vi "UI.vi"() -> ()   [LabVIEW 2016, in "DR803M4.lvlib"]
uses:
  DR803M4.lvlib
  Global variable/hold variable.vi
  Global variable/input variable.vi
  <vilib>/Utility/config.llb/NI_LVConfig.lvlib
panel:
  out "通讯":bool
  out "单次采样量":u16
  out "版本号":string
  out "留样模式":enum16{"定时留样", "时间等比例", "同步留样", "外控留样", "超标留样"}(ring)
  out "门状态":enum16{"门关", "门开"}(ring)
  out "当前瓶号":u16
  out "采样器状态":enum16{"停止", "运行"}(ring)
  out "采样器进程":i32(listbox)
  out "进程":u16(ring) items=["待机"=1, "采样瓶排空"=2, "采样瓶润洗"=5, "进样"=6, "取样"=8, "取样管排空"=9]
  in  "超标留样浓度设置":bool
  out "error out":errorcluster
  in  "VISA资源名称":refnum<visa-resource-name>
  in  "停止":bool
  in  "启动":bool
  in  "门禁":bool
  in  "远程留样":bool
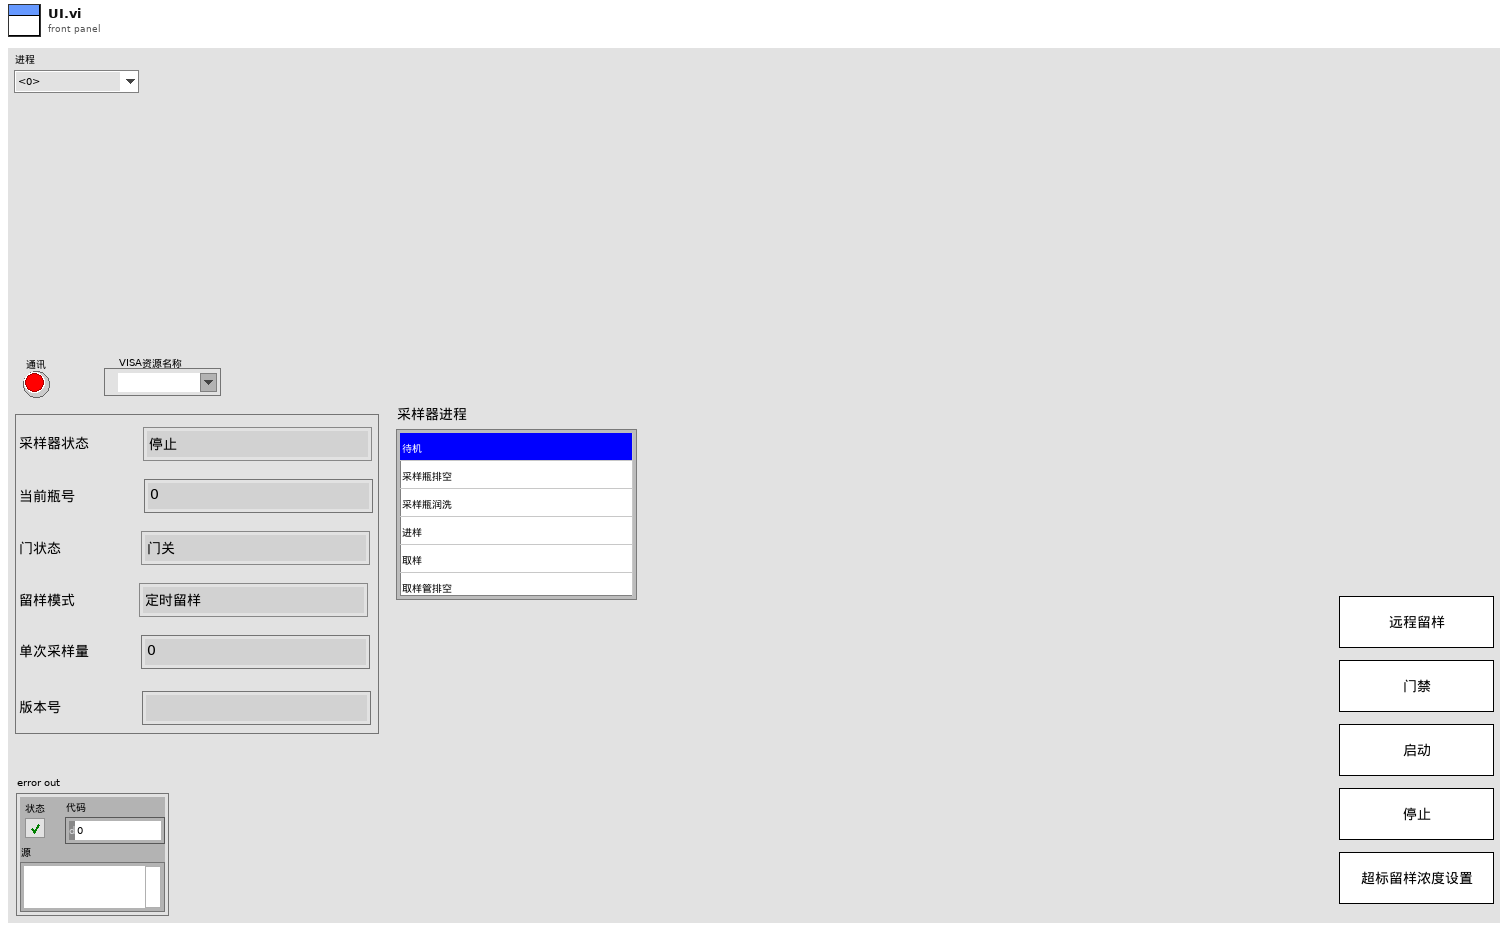
[diagram p1: front panel]
types:
  T1 = cluster{"氨氮超标浓度":dbl, "总磷超标浓度":dbl, "总氮超标浓度":dbl, "CODMn超标浓度":dbl, "CODCr超标浓度":dbl, "PH超标浓度":dbl, "DO超标浓度":dbl, "SPCOND超标浓度":dbl, "浊度超标浓度":dbl, "叶绿素a超标浓度":dbl, "蓝绿藻超标浓度":dbl, "藻密度超标浓度":dbl, "ORP超标浓度":dbl, "COD超标浓度":dbl, "铅超标浓度":dbl, "镉超标浓度":dbl, "铜超标浓度":dbl, "锌超标浓度":dbl, "镍超标浓度":dbl, "锰超标浓度":dbl, "汞超标浓度":dbl}
  T2 = cluster{"确定":bool, "氨氮超标浓度":dbl, "总磷超标浓度":dbl, "总氮超标浓度":dbl, "CODMn超标浓度":dbl, "CODCr超标浓度":dbl, "PH超标浓度":dbl, "DO超标浓度":dbl, "SPCOND超标浓度":dbl, "浊度超标浓度":dbl, "叶绿素a超标浓度":dbl, "蓝绿藻超标浓度":dbl, "藻密度超标浓度":dbl, "ORP超标浓度":dbl, "COD超标浓度":dbl, "铅超标浓度":dbl, "镉超标浓度":dbl, "铜超标浓度":dbl, "锌超标浓度":dbl, "镍超标浓度":dbl, "锰超标浓度":dbl, "汞超标浓度":dbl}
  T3 = typedef "NI_LVConfig.lvlib/Config Data RefNum.ctl" = refnum<k1>
  T4 = cluster{"远程留样":u16, "门禁标志":u16, "门禁密码":u32, "采样器进程":u16, "版本号":string, "启停":u16, "当前瓶号":u16, "采样模式选择":u16, "单次采样量":u16, "时间间隔":u16}
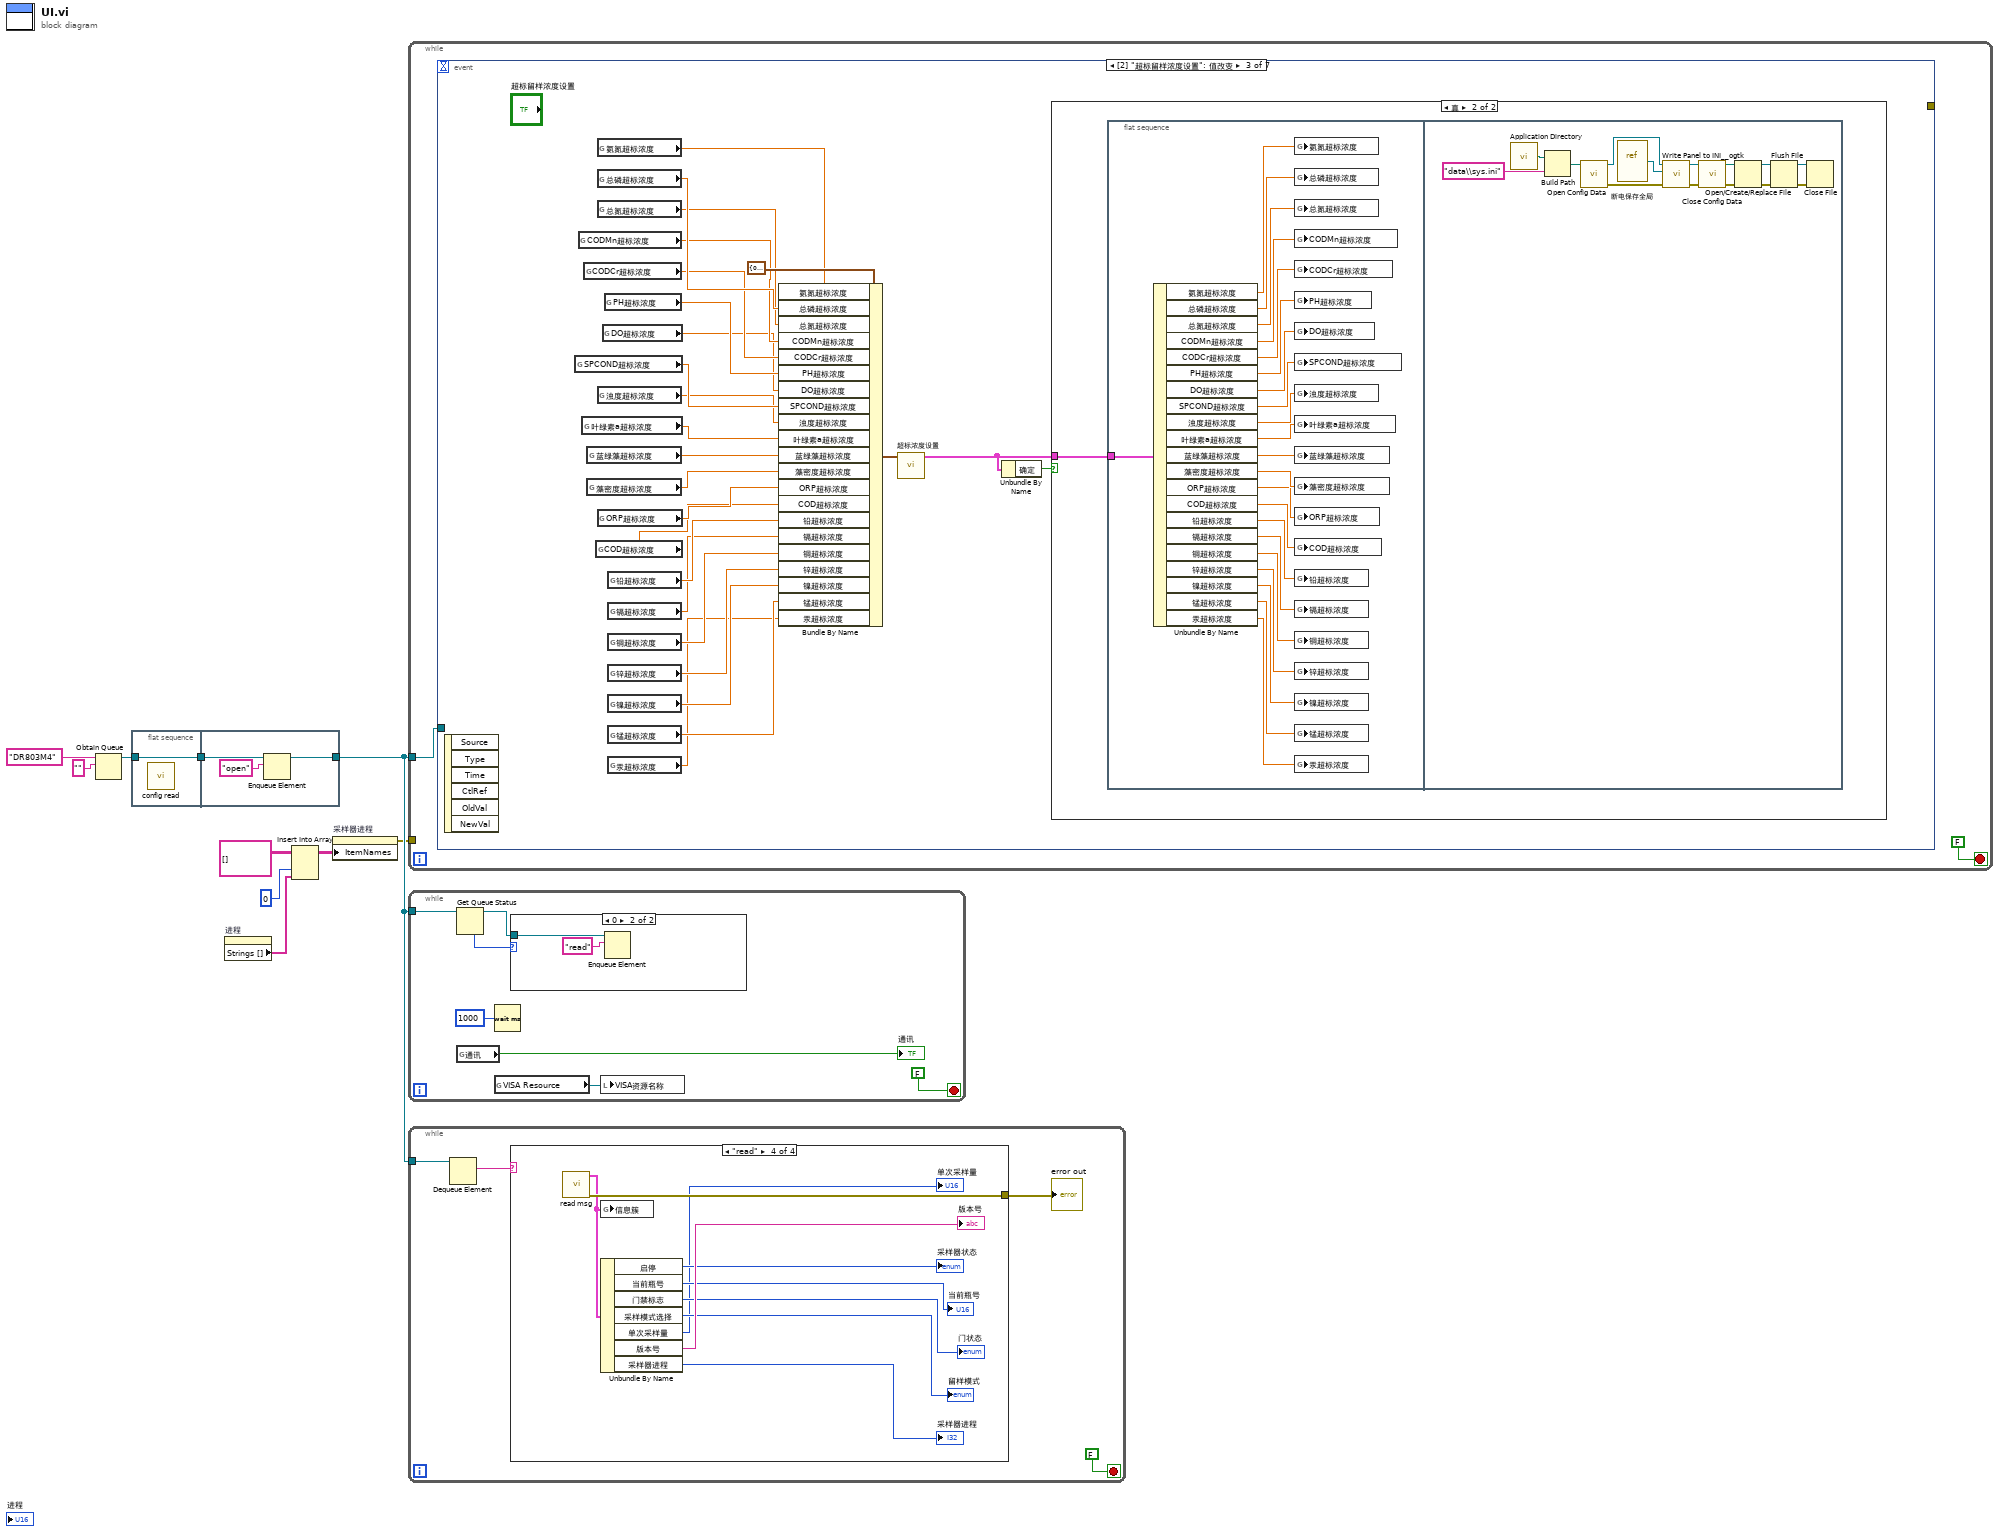
[diagram p0: block diagram]
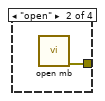
[diagram p4: hidden frame]
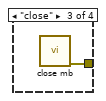
[diagram p5: hidden frame]
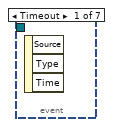
[diagram p6: hidden frame]
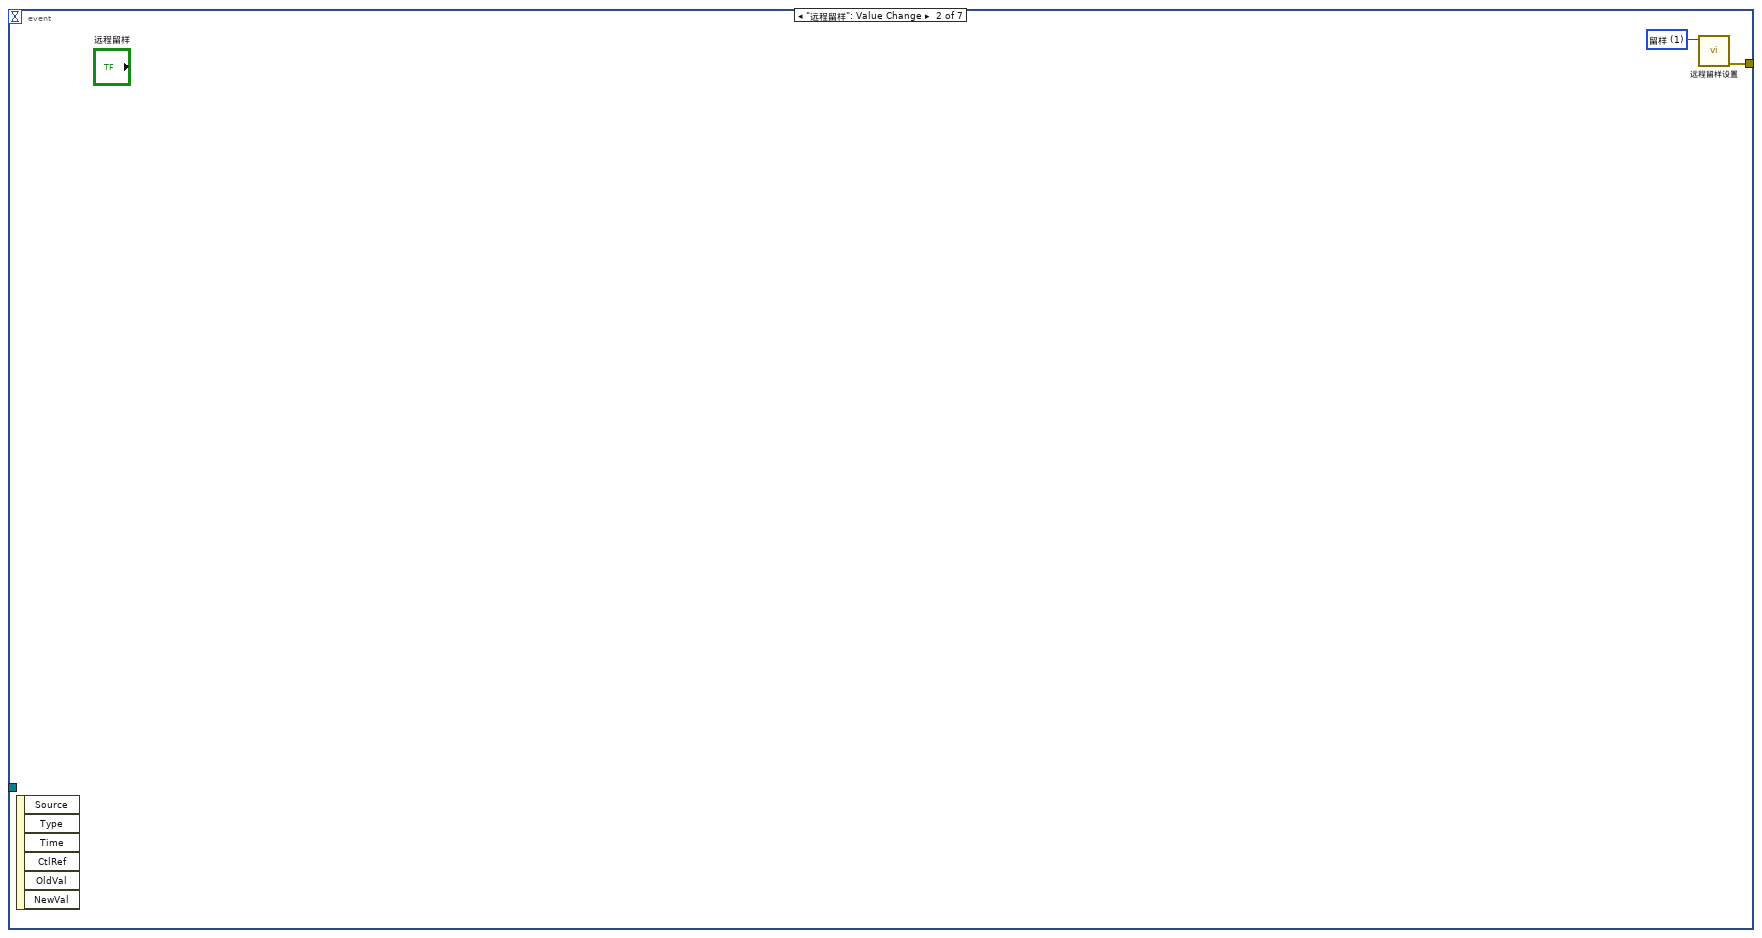
[diagram p7: hidden frame]
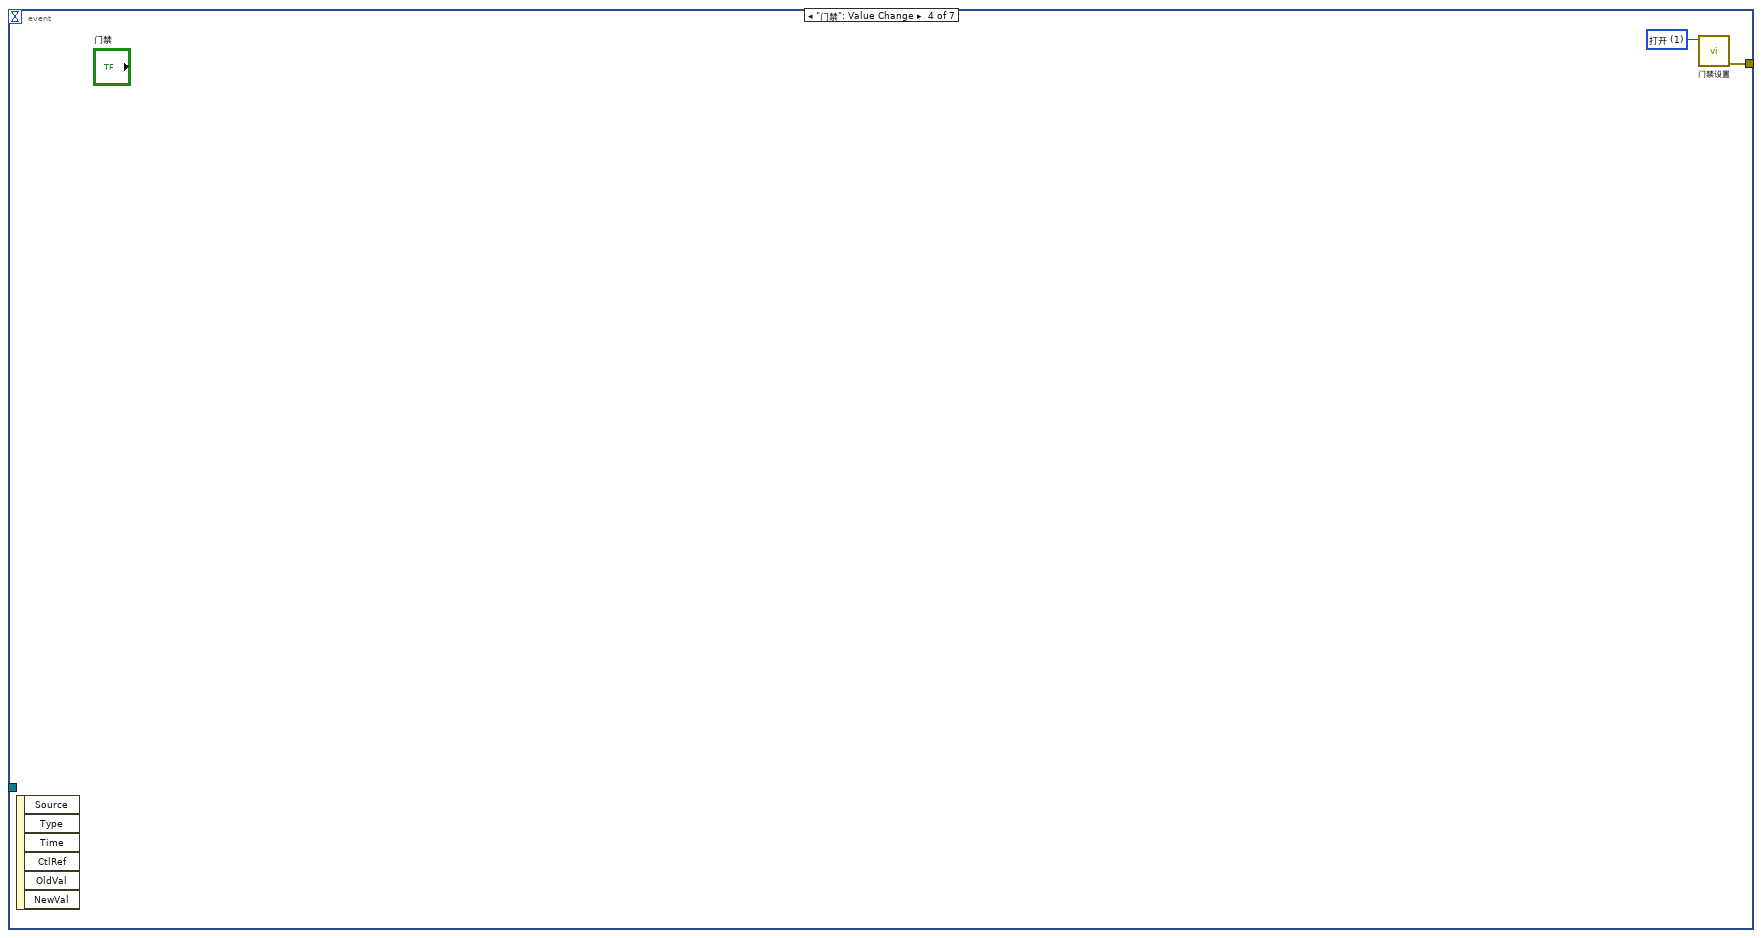
[diagram p9: hidden frame]
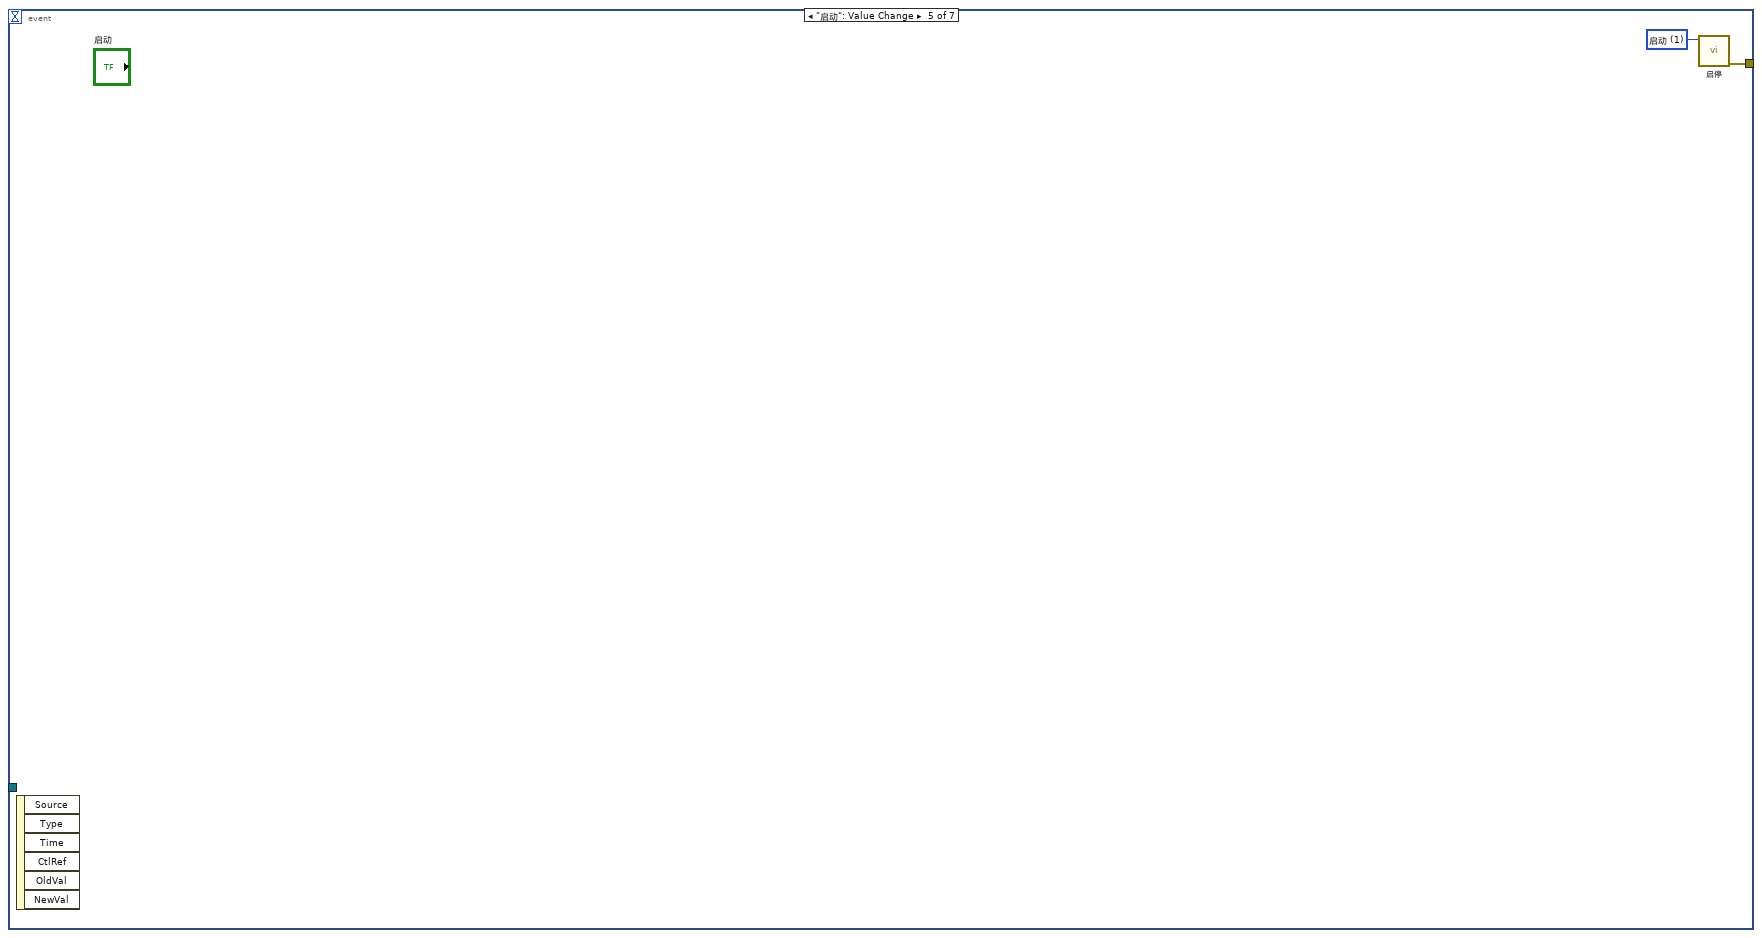
[diagram p10: hidden frame]
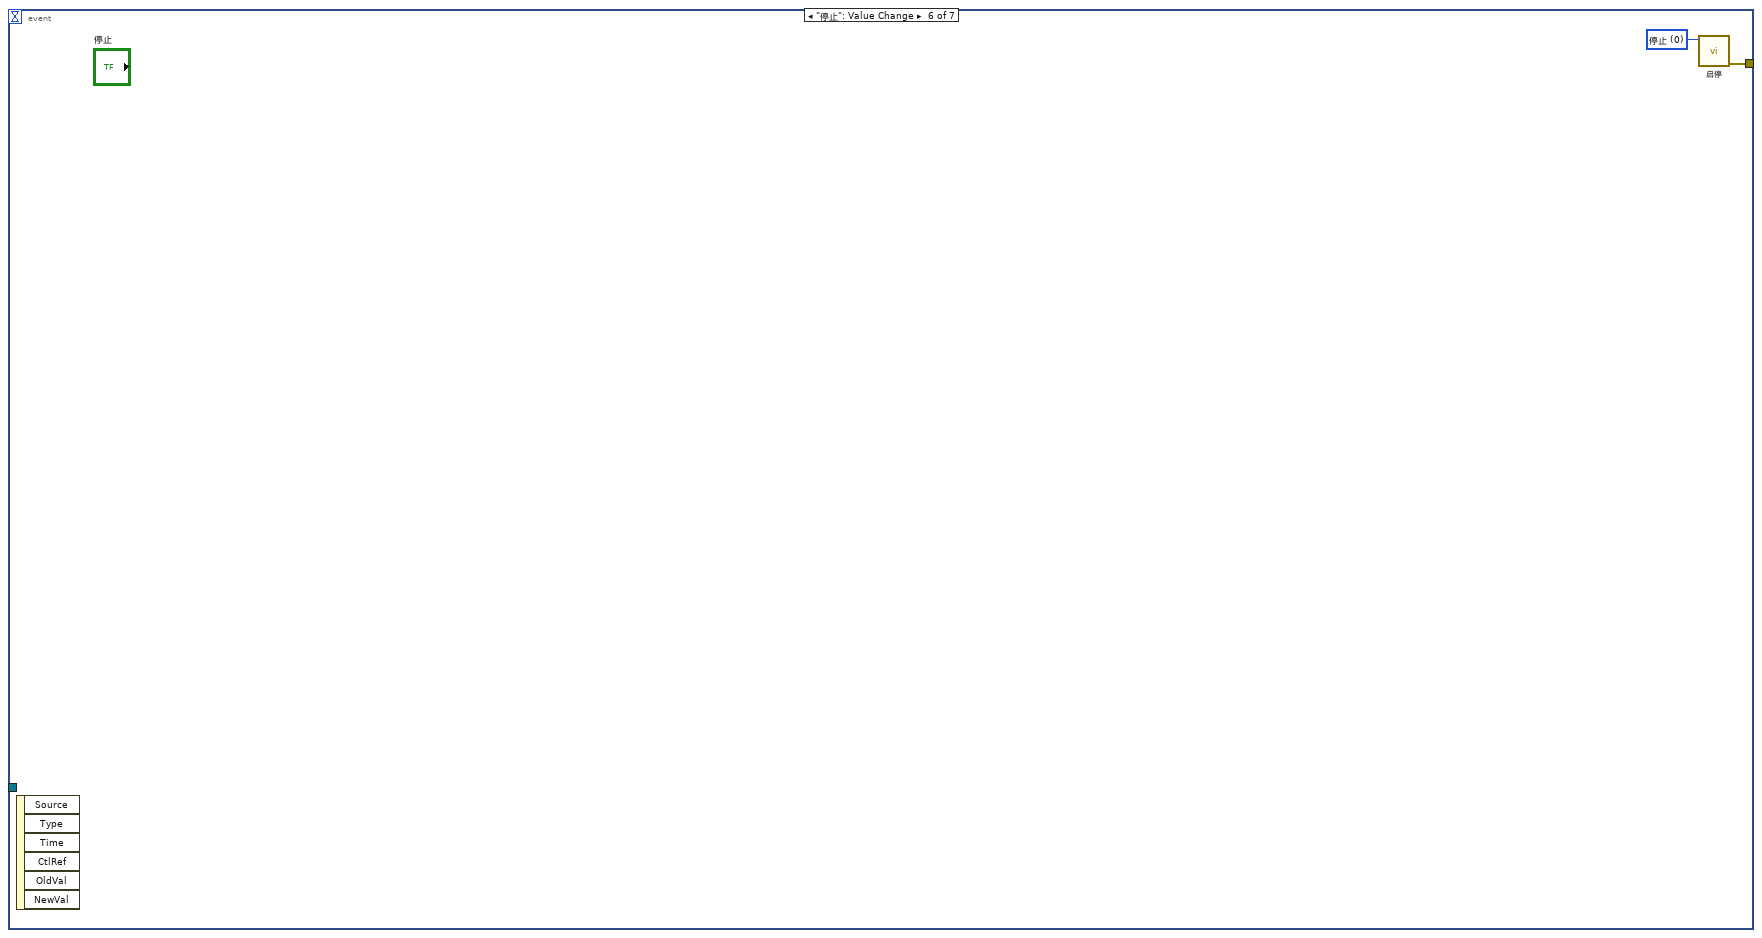
[diagram p11: hidden frame]
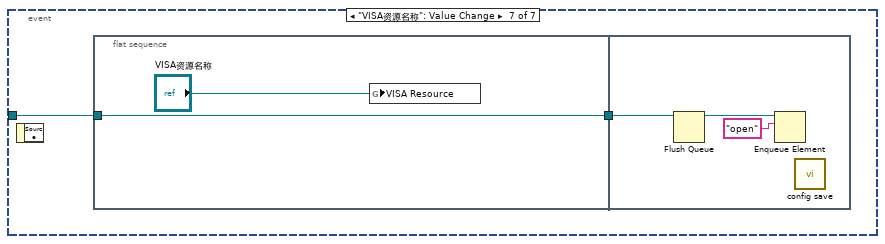
[diagram p12: hidden frame]
diagram:
  n1 = Obtain Queue(name (unnamed)="DR803M4" ("名称（未命名）"), element data type="") -> (queue out=w9:refnum<queue>)  [unwired: 3 in, 2 out]
  n2 = flat-sequence {
    tunnel: w9 -> [w11]
    tunnel: [w11] -> w6
    tunnel: [w13] -> w8
    tunnel: w6 -> [w14]
    frame #0 {
      n3 = call "config read.vi"() -> ()  [unwired: 11 in, 1 out]
    }
    frame #1 {
      n4 = Enqueue Element(queue=w14, element="open" ("元素")) -> (queue out=w13:refnum<queue>)  [unwired: 2 in, 2 out]
    }
  }
  n5 = property on="进程" class="Ring (严格)"() -> ("Strings []"=w3:string[])  [unwired: 2 in, 2 out]
  n6 = Insert Into Array(array=string[][] [] ("字符串[]"), index (col)=0 ("禁用的索引 (列)"), new element=w3) -> (w2:string[][])  [unwired: 1 in]
  n7 = property on="采样器进程" class="MCListbox (严格)"("ItemNames"=w2) -> (error out=w1:errorcluster)  [unwired: 2 in, 1 out]
  n8 = while {
    tunnel: w8 -> [w15]
    tunnel: w1 -> [_]
    stop <- FALSE stop-if-true
    n9 = event shown="[2] \"超标留样浓度设置\": 值改变" {
      selector: _ -> [_ _ _ _ _ _ _]
      dyn-events: _ -> [_ _ _ _ _ _ _]
      timeout: _ -> [_ _ _ _ _ _ _]
      tunnel: [_ w17 _ w81 w84 w86 _] -> _
      tunnel: w15 -> [_ _ _ _ _ _ w87]
      event Timeout {
        n10 = event-data() -> ()  [unwired: 1 in, 3 out]
      }
      event "远程留样": Value Change {
        w18 = u16 1 items=["停止", "留样"] ("远程留样")
        n11 = event-data() -> ()  [unwired: 1 in, 6 out]
        n12 = call "远程留样设置.vi"("远程留样"=w18) -> ("error out"=w17:errorcluster)  [unwired: 10 in]
      }
      event "超标留样浓度设置": Value Change {
        n13 = event-data() -> ()  [unwired: 1 in, 6 out]
        n14 = global read "断电保存全局.vi" "SPCOND超标浓度"() -> (w32:dbl)
        n15 = global read "断电保存全局.vi" "CODMn超标浓度"() -> (w36:dbl)
        n16 = global read "断电保存全局.vi" "叶绿素a超标浓度"() -> (w30:dbl)
        n17 = global read "断电保存全局.vi" "CODCr超标浓度"() -> (w35:dbl)
        n18 = global read "断电保存全局.vi" "蓝绿藻超标浓度"() -> (w29:dbl)
        n19 = global read "断电保存全局.vi" "藻密度超标浓度"() -> (w28:dbl)
        n20 = global read "断电保存全局.vi" "COD超标浓度"() -> (w26:dbl)
        n21 = global read "断电保存全局.vi" "氨氮超标浓度"() -> (w39:dbl)
        n22 = global read "断电保存全局.vi" "总磷超标浓度"() -> (w38:dbl)
        n23 = global read "断电保存全局.vi" "总氮超标浓度"() -> (w37:dbl)
        n24 = global read "断电保存全局.vi" "浊度超标浓度"() -> (w31:dbl)
        n25 = global read "断电保存全局.vi" "ORP超标浓度"() -> (w27:dbl)
        n26 = global read "断电保存全局.vi" "DO超标浓度"() -> (w33:dbl)
        n27 = global read "断电保存全局.vi" "PH超标浓度"() -> (w34:dbl)
        n28 = global read "断电保存全局.vi" "铅超标浓度"() -> (w25:dbl)
        n29 = global read "断电保存全局.vi" "镉超标浓度"() -> (w24:dbl)
        n30 = global read "断电保存全局.vi" "铜超标浓度"() -> (w23:dbl)
        n31 = global read "断电保存全局.vi" "锌超标浓度"() -> (w22:dbl)
        n32 = global read "断电保存全局.vi" "镍超标浓度"() -> (w21:dbl)
        n33 = global read "断电保存全局.vi" "锰超标浓度"() -> (w20:dbl)
        n34 = global read "断电保存全局.vi" "汞超标浓度"() -> (w19:dbl)
        n35 = Bundle By Name(cluster=T1 {"氨氮超标浓度"=0.0, "总磷超标浓度"=0.0, "总氮超标浓度"=0.0, "CODMn超标浓度"=0.0, "CODCr超标浓度"=0.0, "PH超标浓度"=0.0, "DO超标浓度"=0.0, "SPCOND超标浓度"=0.0, "浊度超标浓度"=0.0, "叶绿素a超标浓度"=0.0, "蓝绿藻超标浓度"=0.0, "藻密度超标浓度"=0.0, "ORP超标浓度"=0.0, "COD超标浓度"=0.0, "铅超标浓度"=0.0, "镉超标浓度"=0.0, "铜超标浓度"=0.0, "锌超标浓度"=0.0, "镍超标浓度"=0.0, "锰超标浓度"=0.0, "汞超标浓度"=0.0} ("输入"), "氨氮超标浓度"=w39, "总磷超标浓度"=w38, "总氮超标浓度"=w37, "CODMn超标浓度"=w36, "CODCr超标浓度"=w35, "PH超标浓度"=w34, "DO超标浓度"=w33, "SPCOND超标浓度"=w32, "浊度超标浓度"=w31, "叶绿素a超标浓度"=w30, "蓝绿藻超标浓度"=w29, "藻密度超标浓度"=w28, "ORP超标浓度"=w27, "COD超标浓度"=w26, "铅超标浓度"=w25, "镉超标浓度"=w24, "铜超标浓度"=w23, "锌超标浓度"=w22, "镍超标浓度"=w21, "锰超标浓度"=w20, "汞超标浓度"=w19) -> (w41:T1)
        n36 = call "超标浓度设置.vi"("输入"=w41) -> ("输出"=w42:T2)  [unwired: 10 in]
        n37 = Unbundle By Name(w42) -> ("确定"=w43:bool)
        n38 = case shown="真" w43 {
          tunnel: w42 -> [_ w44]
          frame False {
          }
          frame True {
            n39 = flat-sequence {
              tunnel: w44 -> [w66]
              frame #0 {
                n40 = Unbundle By Name(w66) -> ("氨氮超标浓度"=w65:dbl, "总磷超标浓度"=w64:dbl, "总氮超标浓度"=w63:dbl, "CODMn超标浓度"=w62:dbl, "CODCr超标浓度"=w61:dbl, "PH超标浓度"=w60:dbl, "DO超标浓度"=w59:dbl, "SPCOND超标浓度"=w58:dbl, "浊度超标浓度"=w57:dbl, "叶绿素a超标浓度"=w56:dbl, "蓝绿藻超标浓度"=w55:dbl, "藻密度超标浓度"=w54:dbl, "ORP超标浓度"=w53:dbl, "COD超标浓度"=w52:dbl, "铅超标浓度"=w51:dbl, "镉超标浓度"=w50:dbl, "铜超标浓度"=w49:dbl, "锌超标浓度"=w48:dbl, "镍超标浓度"=w47:dbl, "锰超标浓度"=w46:dbl, "汞超标浓度"=w45:dbl)
                n41 = global write "断电保存全局.vi" "氨氮超标浓度"(w65) -> ()
                n42 = global write "断电保存全局.vi" "总磷超标浓度"(w64) -> ()
                n43 = global write "断电保存全局.vi" "总氮超标浓度"(w63) -> ()
                n44 = global write "断电保存全局.vi" "CODMn超标浓度"(w62) -> ()
                n45 = global write "断电保存全局.vi" "CODCr超标浓度"(w61) -> ()
                n46 = global write "断电保存全局.vi" "PH超标浓度"(w60) -> ()
                n47 = global write "断电保存全局.vi" "DO超标浓度"(w59) -> ()
                n48 = global write "断电保存全局.vi" "SPCOND超标浓度"(w58) -> ()
                n49 = global write "断电保存全局.vi" "浊度超标浓度"(w57) -> ()
                n50 = global write "断电保存全局.vi" "叶绿素a超标浓度"(w56) -> ()
                n51 = global write "断电保存全局.vi" "蓝绿藻超标浓度"(w55) -> ()
                n52 = global write "断电保存全局.vi" "藻密度超标浓度"(w54) -> ()
                n53 = global write "断电保存全局.vi" "ORP超标浓度"(w53) -> ()
                n54 = global write "断电保存全局.vi" "COD超标浓度"(w52) -> ()
                n55 = global write "断电保存全局.vi" "铅超标浓度"(w51) -> ()
                n56 = global write "断电保存全局.vi" "镉超标浓度"(w50) -> ()
                n57 = global write "断电保存全局.vi" "铜超标浓度"(w49) -> ()
                n58 = global write "断电保存全局.vi" "锌超标浓度"(w48) -> ()
                n59 = global write "断电保存全局.vi" "镍超标浓度"(w47) -> ()
                n60 = global write "断电保存全局.vi" "锰超标浓度"(w46) -> ()
                n61 = global write "断电保存全局.vi" "汞超标浓度"(w45) -> ()
              }
              frame #1 {
                n62 = call <vilib>:"Application Directory.vi"() -> ("Application Directory"=w79:path)
                n63 = Build Path(base path=w79, name or relative path="data\\sys.ini" ("名称或相对路径")) -> (appended path=w78:path)
                n64 = call <vilib>:"Open Config Data.vi"("configuration file path"=w78) -> ("error out"=w74:errorcluster, "refnum"=w77:T3)  [unwired: 8 in, 1 out]
                n65 = vi-ref "断电保存全局.vi"() -> (w76:refnum<vi>)
                n66 = call <userlib>:"Write Panel to INI__ogtk.vi"("error in (no error)"=w74, "VI ref"=w76, "refnum"=w77) -> ("error out"=w73:errorcluster, "refnum out"=w75:T3)  [unwired: 7 in]
                n67 = call <vilib>:"Close Config Data.vi"("error in (no error)"=w73, "refnum"=w75) -> ("error out"=w68:errorcluster, "file path"=w67:path)  [unwired: 8 in]
                n68 = Open/Create/Replace File(file path (use dialog)=w67, error in=w68) -> (refnum out=w71:refnum<file>, error out=w72:errorcluster)  [unwired: 4 in, 1 out]
                n69 = Flush File(refnum=w71, error in=w72) -> (refnum out=w70:refnum<file>, error out=w69:errorcluster)
                n70 = Close File(refnum=w70, error in=w69) -> ()  [unwired: 2 out]
              }
            }
          }
        }
      }
      event "门禁": Value Change {
        w82 = u16 1 items=["关闭", "打开"] ("门禁标志")
        n71 = event-data() -> ()  [unwired: 1 in, 6 out]
        n72 = call "门禁设置.vi"("门禁标志"=w82) -> ("error out"=w81:errorcluster)  [unwired: 10 in]
      }
      event "启动": Value Change {
        w83 = u16 1 items=["停止", "启动"] ("启停")
        n73 = event-data() -> ()  [unwired: 1 in, 6 out]
        n74 = call "启停.vi"("启停"=w83) -> ("error out"=w84:errorcluster)  [unwired: 10 in]
      }
      event "停止": Value Change {
        w85 = u16 0 items=["停止", "启动"] ("启停")
        n75 = event-data() -> ()  [unwired: 1 in, 6 out]
        n76 = call "启停.vi"("启停"=w85) -> ("error out"=w86:errorcluster)  [unwired: 10 in]
      }
      event "VISA资源名称": Value Change {
        n77 = event-data() -> ()  [unwired: 1 in, 1 out]
        n78 = flat-sequence {
          tunnel: [w89] -> w88
          tunnel: w87 -> [w89]
          tunnel: w88 -> [w92]
          frame #0 {
            n79 = global write "hold variable.vi" "VISA Resource"("VISA资源名称") -> ()
          }
          frame #1 {
            n80 = Flush Queue(queue=w92) -> (queue out=w93:refnum<queue>)  [unwired: 1 in, 2 out]
            n81 = Enqueue Element(queue=w93, element="open" ("元素")) -> ()  [unwired: 2 in, 3 out]
            n82 = call "config save.vi"() -> ()  [unwired: 11 in, 1 out]
          }
        }
      }
    }
  }
  n83 = while {
    tunnel: w8 -> [w97]
    stop <- FALSE stop-if-true
    n84 = Get Queue Status(queue=w97) -> (queue out=w95:refnum<queue>, # elements in queue=w96:i32)  [unwired: 2 in, 6 out]
    n85 = global read "hold variable.vi" "通讯"() -> (→"通讯":bool)
    n86 = Wait (ms)(milliseconds to wait=u32 1000 ("等待时间（毫秒）")) -> ()  [unwired: 1 out]
    n87 = global read "hold variable.vi" "VISA Resource"() -> (w98:refnum<visa-resource-name>)
    n88 = case shown="0" w96 {
      tunnel: w95 -> [_ w102]
      frame Default {
      }
      frame 0 {
        n89 = Enqueue Element(queue=w102, element="read" ("元素")) -> ()  [unwired: 2 in, 3 out]
      }
    }
    n90 = local write "VISA资源名称"(w98) -> ()
  }
  n91 = while {
    tunnel: w8 -> [w106]
    stop <- FALSE stop-if-true
    n92 = Dequeue Element(queue=w106) -> (element=w105:string)  [unwired: 2 in, 3 out]
    n93 = case shown="\"read\"" w105 {
      tunnel: [_ w107 w108 w117] -> w104
      frame Default {
      }
      frame "open" {
        n94 = call "open mb.vi"() -> ("Error out"=w107:errorcluster)  [unwired: 11 in]
      }
      frame "close" {
        n95 = call "close mb.vi"() -> ("error out"=w108:errorcluster)  [unwired: 11 in]
      }
      frame "read" {
        n96 = call "read msg.vi"() -> ("error out"=w117:errorcluster, "信息簇"=w116:T4)  [unwired: 10 in]
        n97 = global write "input variable.vi" "信息簇"(w116) -> ()
        n98 = Unbundle By Name(w116) -> ("启停"=→"采样器状态":u16, "当前瓶号"=→"当前瓶号":u16, "门禁标志"=→"门状态":u16, "采样模式选择"=→"留样模式":u16, "单次采样量"=→"单次采样量":u16, "版本号"=→"版本号":string, "采样器进程"=→"采样器进程":u16)
      }
    }
    "error out" <- w104
  }
